vi "Blink3LED.vi"() -> ()   [LabVIEW 2015]
panel:
  out "LED2V":bool
  in  "LED2":bool
  out "YLDRMErrorOut":errorcluster
  in  "YLDRMPortInp":refnum<visa-resource-name>
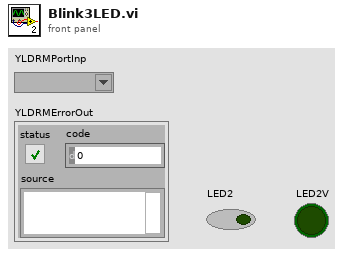
[diagram p1: front panel]
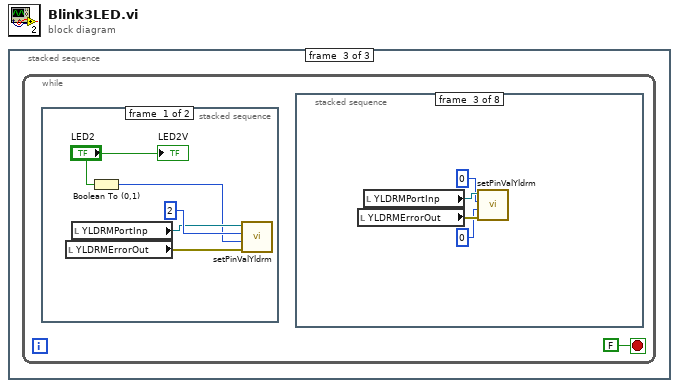
[diagram p0: block diagram]
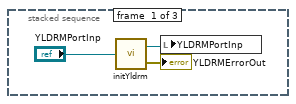
[diagram p2: hidden frame]
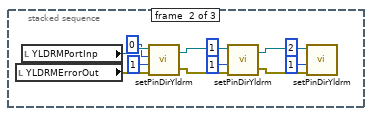
[diagram p3: hidden frame]
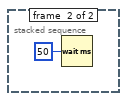
[diagram p4: hidden frame]
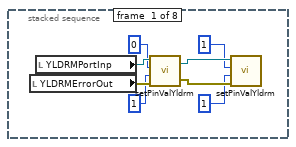
[diagram p5: hidden frame]
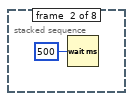
[diagram p6: hidden frame]
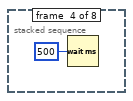
[diagram p7: hidden frame]
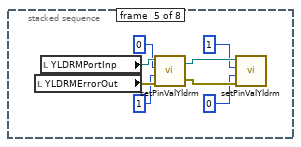
[diagram p8: hidden frame]
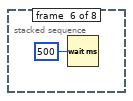
[diagram p9: hidden frame]
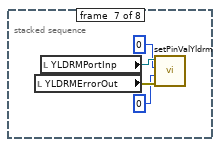
[diagram p10: hidden frame]
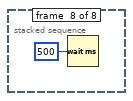
[diagram p11: hidden frame]
diagram:
  n1 = stacked-sequence {
    frame #0 {
      n2 = call "initYldrm.vi"("YLDRMPortInp"="YLDRMPortInp") -> ("YLDRMPortOut"=w2:refnum<visa-resource-name>, "YLDRMErrorOut"=→"YLDRMErrorOut":errorcluster)
      n3 = local write "YLDRMPortInp"(w2) -> ()
    }
    frame #1 {
      n4 = local read "YLDRMErrorOut"() -> (w14:errorcluster)
      n5 = local read "YLDRMPortInp"() -> (w15:refnum<visa-resource-name>)
      n6 = call "setPinDirYldrm.vi"("YLDRMErrorInp"=w14, "dir"=u8 1, "pin"=u8 0, "YLDRMPortInp"=w15) -> ("YLDRMErrorOut"=w13:errorcluster, "YLDRMPortOut"=w11:refnum<visa-resource-name>)
      n7 = call "setPinDirYldrm.vi"("YLDRMErrorInp"=w13, "dir"=u8 1, "pin"=u8 1, "YLDRMPortInp"=w11) -> ("YLDRMErrorOut"=w12:errorcluster, "YLDRMPortOut"=w10:refnum<visa-resource-name>)
      n8 = call "setPinDirYldrm.vi"("YLDRMErrorInp"=w12, "dir"=u8 1, "pin"=u8 2, "YLDRMPortInp"=w10) -> ()  [unwired: 2 out]
    }
    frame #2 {
      n9 = while {
        stop <- FALSE stop-if-true
        n10 = stacked-sequence {
          frame #0 {
            n11 = local read "YLDRMErrorOut"() -> (w19:errorcluster)
            n12 = local read "YLDRMPortInp"() -> (w20:refnum<visa-resource-name>)
            n13 = Boolean To (0,1)(Boolean="LED2") -> (0, 1=w17:i16)
            n14 = call "setPinValYldrm.vi"("YLDRMErrorInp"=w19, "val"=w17, "pin"=u8 2, "YLDRMPortInp"=w20) -> ()  [unwired: 2 out]
            "LED2V" <- "LED2"
          }
          frame #1 {
            n15 = Wait (ms)(milliseconds to wait=u32 50) -> ()  [unwired: 1 out]
          }
        }
        n16 = stacked-sequence {
          frame #0 {
            n17 = local read "YLDRMErrorOut"() -> (w30:errorcluster)
            n18 = local read "YLDRMPortInp"() -> (w29:refnum<visa-resource-name>)
            n19 = call "setPinValYldrm.vi"("YLDRMErrorInp"=w30, "val"=u8 1, "pin"=u8 0, "YLDRMPortInp"=w29) -> ("YLDRMErrorOut"=w25:errorcluster, "YLDRMPortOut"=w26:refnum<visa-resource-name>)
            n20 = call "setPinValYldrm.vi"("YLDRMErrorInp"=w25, "val"=u8 1, "pin"=u8 1, "YLDRMPortInp"=w26) -> ()  [unwired: 2 out]
          }
          frame #1 {
            n21 = Wait (ms)(milliseconds to wait=u32 500) -> ()  [unwired: 1 out]
          }
          frame #2 {
            n22 = local read "YLDRMErrorOut"() -> (w35:errorcluster)
            n23 = local read "YLDRMPortInp"() -> (w34:refnum<visa-resource-name>)
            n24 = call "setPinValYldrm.vi"("YLDRMErrorInp"=w35, "val"=u8 0, "pin"=u8 0, "YLDRMPortInp"=w34) -> ()  [unwired: 2 out]
          }
          frame #3 {
            n25 = Wait (ms)(milliseconds to wait=u32 500) -> ()  [unwired: 1 out]
          }
          frame #4 {
            n26 = local read "YLDRMErrorOut"() -> (w44:errorcluster)
            n27 = local read "YLDRMPortInp"() -> (w43:refnum<visa-resource-name>)
            n28 = call "setPinValYldrm.vi"("YLDRMErrorInp"=w44, "val"=u8 1, "pin"=u8 0, "YLDRMPortInp"=w43) -> ("YLDRMErrorOut"=w39:errorcluster, "YLDRMPortOut"=w40:refnum<visa-resource-name>)
            n29 = call "setPinValYldrm.vi"("YLDRMErrorInp"=w39, "val"=u8 0, "pin"=u8 1, "YLDRMPortInp"=w40) -> ()  [unwired: 2 out]
          }
          frame #5 {
            n30 = Wait (ms)(milliseconds to wait=u32 500) -> ()  [unwired: 1 out]
          }
          frame #6 {
            n31 = local read "YLDRMErrorOut"() -> (w49:errorcluster)
            n32 = local read "YLDRMPortInp"() -> (w48:refnum<visa-resource-name>)
            n33 = call "setPinValYldrm.vi"("YLDRMErrorInp"=w49, "val"=u8 0, "pin"=u8 0, "YLDRMPortInp"=w48) -> ()  [unwired: 2 out]
          }
          frame #7 {
            n34 = Wait (ms)(milliseconds to wait=u32 500) -> ()  [unwired: 1 out]
          }
        }
      }
    }
  }
